vi "SLL Easy API Server Example.vi"() -> ()   [LabVIEW 2016, in "SLL Easy API via TCP.lvclass"]
uses:
  SLL Easy API via TCP.lvclass
  _SubVIs/TCP Initialize Server - Local.vi
panel:
  out "error out":errorcluster
  out "Last Received Response":string
  in  "Exit":bool
  in  "Service Name":string="SLL Easy TCP Service"
  # "After running this VI, run the Client Write or Write Read Example"
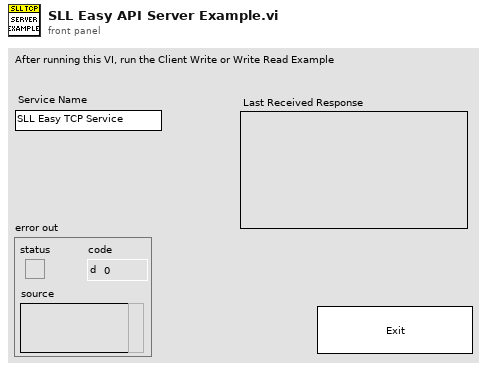
[diagram p1: front panel]
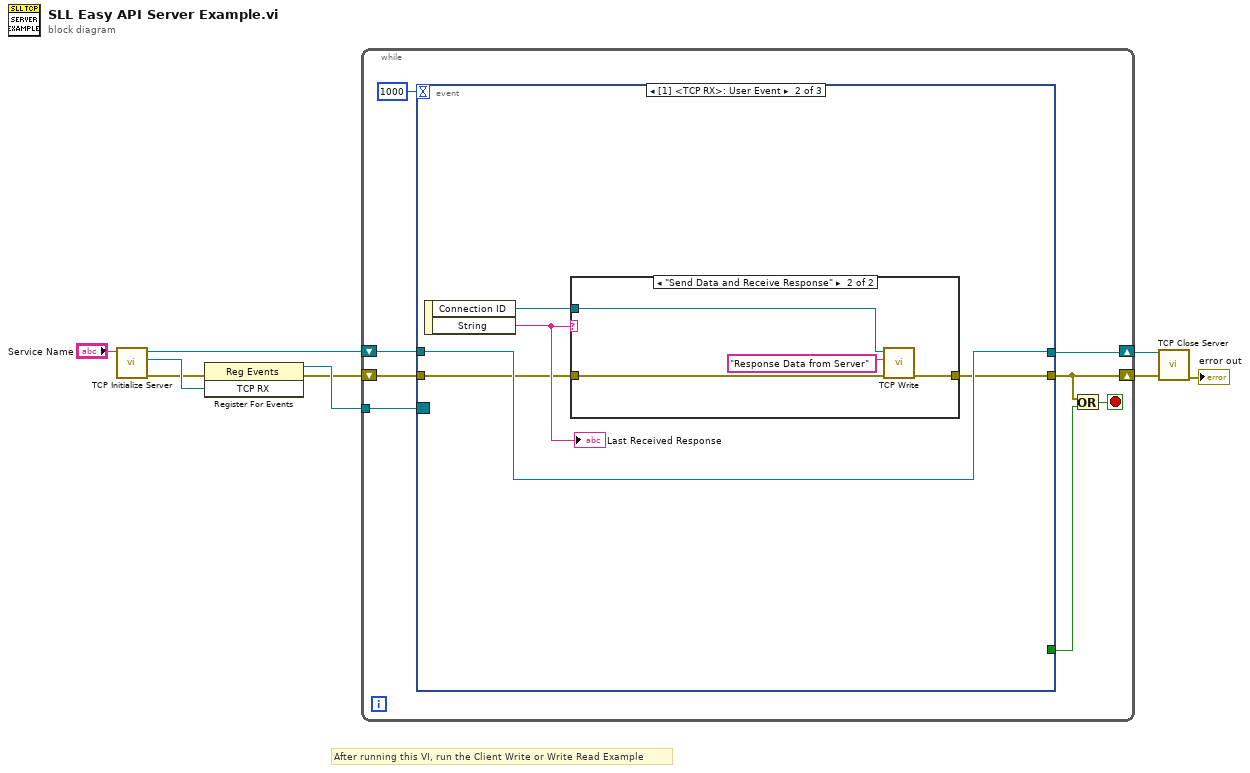
[diagram p0: block diagram]
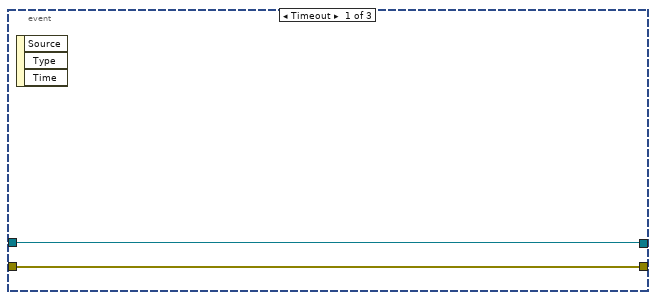
[diagram p2: hidden frame]
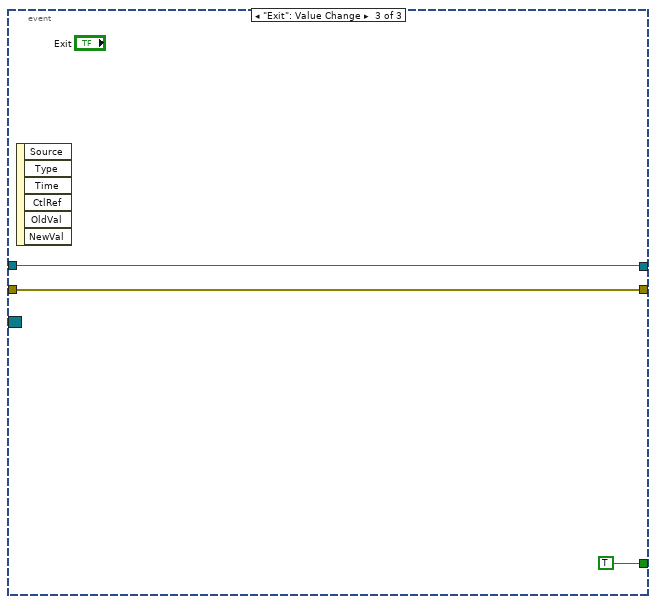
[diagram p4: hidden frame]
diagram:
  # "After running this VI, run the Client Write or Write Read Example"
  n1 = call-poly "TCP Initialize Server.vi"("Service Name"="Service Name") -> ("error out"=w4:errorcluster, "TCP RX"=w7:refnum<user-event>, "SLL Easy API via TCP out"=w8:refnum<class "SLL Easy API via TCP.lvclass">)  [unwired: 8 in]
  n2 = register-events(error in=w4, w7) -> (reference out=w6:refnum<event-registration>, error out=w3:errorcluster)  [unwired: 1 in]
  n3 = while {
    tunnel: w6 -> [w17]
    shift-right: [w12] -> w2
    shift-left: w3 -> [w13]
    shift-right: [w15] -> w5
    shift-left: w8 -> [w14]
    stop <- w10 stop-if-true
    n4 = event shown="[1] <TCP RX>: User Event" {
      selector: w17 -> [_ _ _]
      dyn-events: _ -> [_ _ _]
      timeout: 1000 -> [_ _ _]
      tunnel: [w19 w24 w32] -> w15
      tunnel: w14 -> [w19 w24 w32]
      tunnel: [_ _ TRUE] -> w11
      tunnel: w13 -> [w18 w21 w30]
      tunnel: [w18 w20 w30] -> w12
      event Timeout {
        n5 = event-data() -> ()  [unwired: 1 in, 3 out]
      }
      event User Event {
        n6 = event-data() -> ("Connection ID"=w22:refnum<k5>, "String"=w23:string)  [unwired: 1 in]
        "Last Received Response" <- w23
        n7 = case shown="\"Send Data and Receive Response\"" w23 {
          tunnel: w22 -> [_ w29]
          tunnel: w21 -> [w25 w27]
          tunnel: [w25 w26] -> w20
          frame Default {
          }
          frame "Send Data and Receive Response" {
            n8 = call "TCP Write.vi"("error in (no error)"=w27, "Write Data"="Response Data from Server", "connection ID In"=w29) -> ("error out"=w26:errorcluster)  [unwired: 7 in, 1 out]
          }
        }
      }
      event "Exit": Value Change {
        n9 = event-data() -> ()  [unwired: 1 in, 6 out]
      }
    }
    n10 = Or(x=w12, y=w11) -> (x .or. y?=w10:bool)
  }
  n11 = call "TCP Close Server.vi"("error in (no error)"=w2, "SLL Easy API via TCP in"=w5) -> ("error out"=→"error out":errorcluster)  [unwired: 9 in]
